vi "Get Measurement Details.vi"(8 "error in":errorcluster) -> (0 "error out":errorcluster, 2 "Service Class":string, 3 "Measurement Details":T1)   [LabVIEW 2023, in "LabVIEW Bodeplot Summit.lvlib"]
uses:
  LabVIEW Bodeplot Summit.lvlib
  <vilib>/MeasurementLink/MeasurementLink Measurement Server Internal/RPC Messages/ni_measurementlink_measurement_v1_MeasurementDetails.ctl
  <vilib>/MeasurementLink/MeasurementLink Measurement Server Internal/MeasurementLink Measurement Server Internal.lvlib
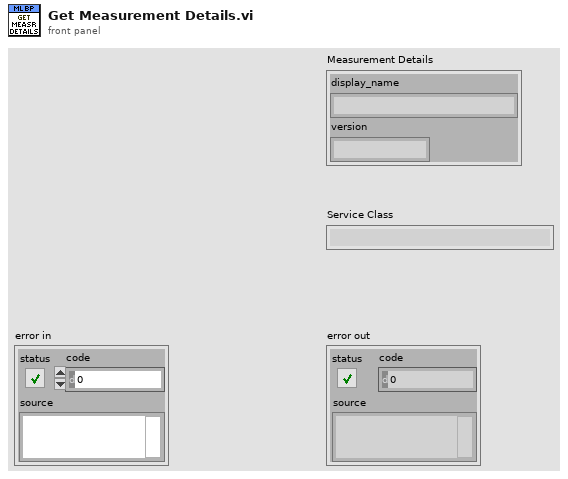
[diagram p1: front panel]
types:
  T1 = typedef "MeasurementLink Measurement Server Internal.lvlib/ni_measurementlink_measurement_v1_MeasurementDetails.ctl" = cluster{"display_name":string, "version":string}
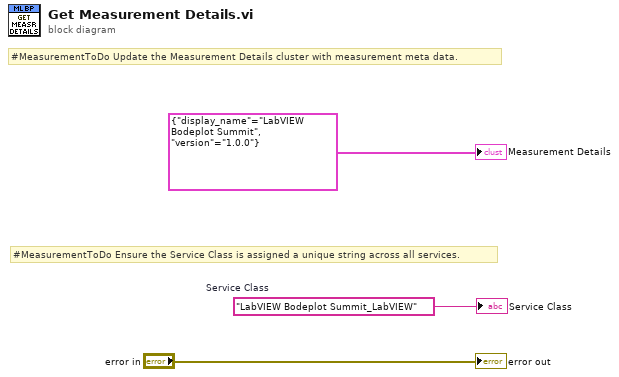
[diagram p0: block diagram]
diagram:
  w2 = "LabVIEW Bodeplot Summit_LabVIEW"  # Service Class
  # "#MeasurementToDo Ensure the Service Class is assigned a unique string across all services."
  # "#MeasurementToDo Update the Measurement Details cluster with measurement meta data."
  "error out" <- "error in"
  "Measurement Details" <- T1 {"display_name"="LabVIEW Bodeplot Summit", "version"="1.0.0"} ("Measurement Details")
  "Service Class" <- w2
